vi "New Connection Listener.vi"(7 "Connection Listener in":refnum<class "Connection Listener.lvclass">, 8 "error in (no error)":errorcluster, 11 "Port":u16) -> (0 "error out":errorcluster, 3 "Connection Listener out":refnum<class "Connection Listener.lvclass">)   [LabVIEW 2017, in "Connection Listener.lvlib" / "Connection Listener.lvclass"]
uses:
  Connection Listener.lvclass
  Connection Listener.lvclass/Connection Listener.ctl
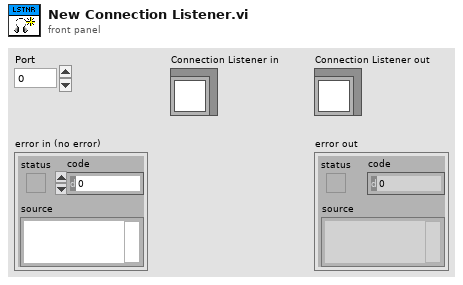
[diagram p1: front panel]
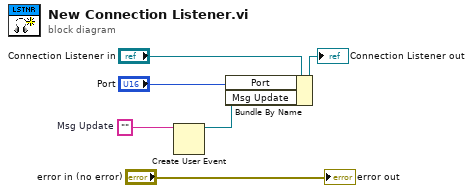
[diagram p0: block diagram]
diagram:
  w1 = ""  # Msg Update
  n1 = Create User Event(user event datatype=w1) -> (user event=w2:refnum<user-event>)  [unwired: 1 in, 1 out]
  n2 = Bundle By Name(cluster="Connection Listener in", "Port"="Port", "Msg Update"=w2) -> (→"Connection Listener out":refnum<class "Connection Listener.lvclass">)
  "error out" <- "error in (no error)"
